vi "outgoing data.vi"(6 "timeout (-1)":i32=-1, 8 "error in":errorcluster, 11 "Websocket console plugin in":refnum<class "Websocket console plugin.lvclass">) -> (0 "error out":errorcluster, 1 "timeout":bool, 2 "opcode":u8=1, 3 "data":string, 5 "not last fragment (F)":bool, 7 "kill connection":bool)   [LabVIEW 2016, in "Websocket console plugin.lvclass"]
uses:
  Websocket console plugin.lvclass
  websocket/opcode.ctl
  Websocket console plugin.lvclass/Websocket console plugin.ctl
  websocket/websocket core.lvlib
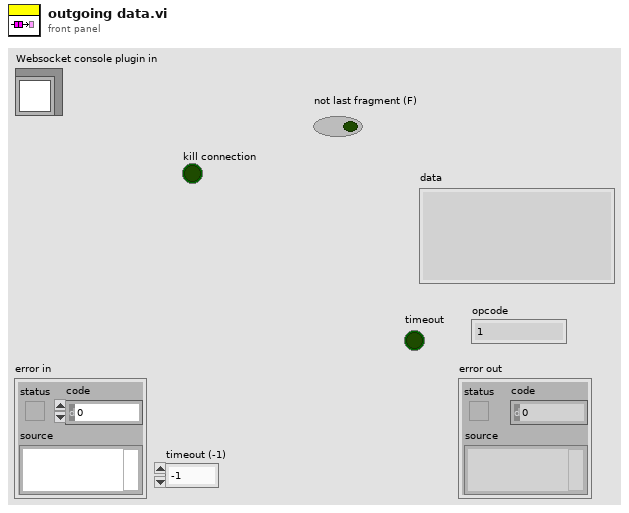
[diagram p1: front panel]
types:
  T1 = typedef "websocket core.lvlib/opcode.ctl" = u8
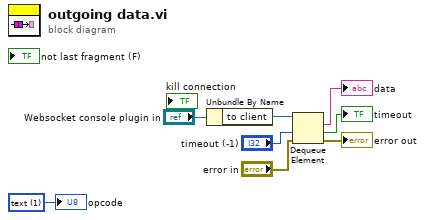
[diagram p0: block diagram]
diagram:
  w2 = T1 1 items=["text"=1, "binary"=2, "x3"=3, "x4"=4, "x5"=5, "x6"=6, "x7"=7] ("opcode")
  n1 = Unbundle By Name("Websocket console plugin in") -> ("to client"=w4:refnum<queue>)
  n2 = Dequeue Element(queue=w4, timeout in ms (-1)="timeout (-1)", error in (no error)="error in") -> (element=→"data":string, timed out?=→"timeout":bool, error out=→"error out":errorcluster)  [unwired: 1 out]
  "opcode" <- w2
